vi "TL behavior obstacle avoidance.vi"(1 "Activate?":bool=TRUE, 2 "Sensor":cluster{"Name":string, "f":dbl}[](array[cluster])=[{"Name"="bow", "f"=20.0}, {"Name"="pbow", "f"=60.0}, {"Name"="port", "f"=0.0}, {"Name"="sbow", "f"=60.0}, {"Name"="starboard", "f"=0.0}]) -> (0 "Obs Avoid Array":dbl[](array[numeric]))   [LabVIEW 2013]
doc: "This vi uses the values from the Bow, PBow and SBow IR sensors to create an Obstacle Avoidance Array. The value range between 1 and -1."
panel:
  out "Waveform Graph":cluster{dbl, dbl, dbl[]}(graph)
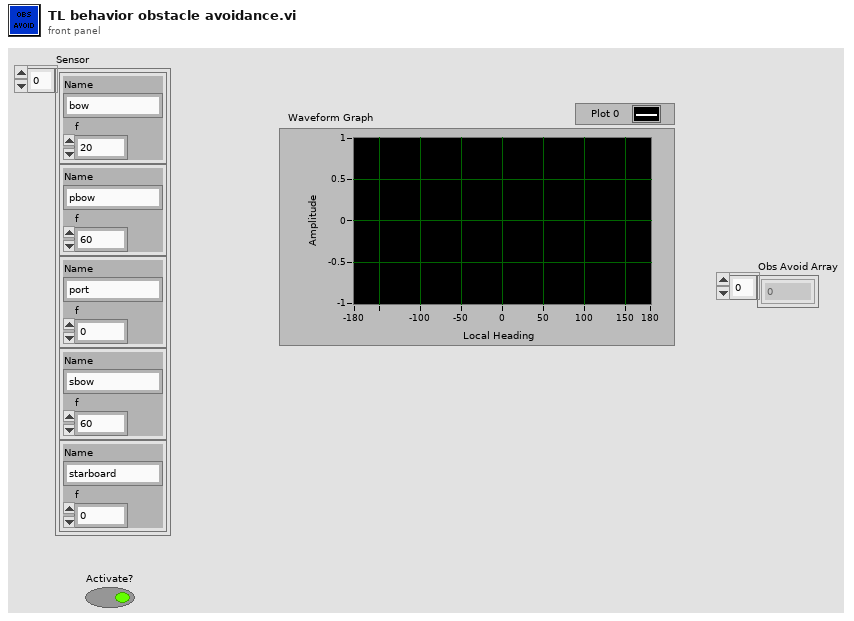
[diagram p1: front panel]
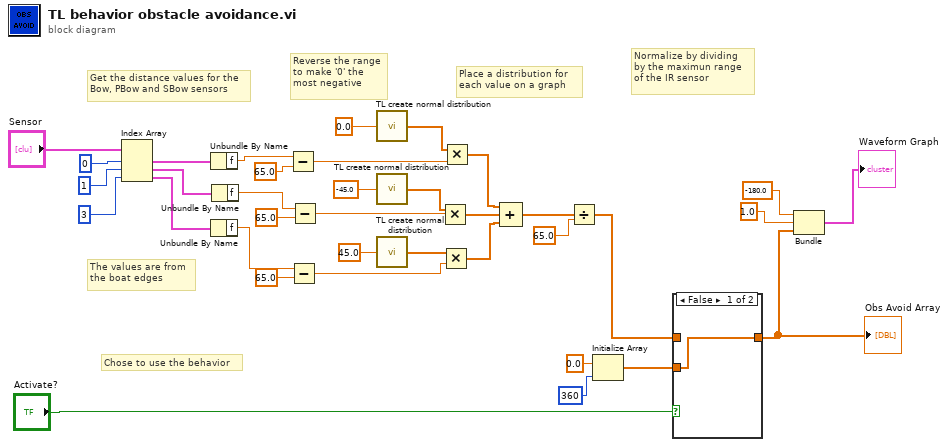
[diagram p0: block diagram]
diagram:
  # "Chose to use the behavior"
  # "Reverse the range\nto make '0' the\nmost negative"
  # "Normalize by dividing\nby the maximun range\nof the IR sensor"
  # "The values are from\nthe boat edges"
  # "Place a distribution for \neach value on a graph"
  # "Get the distance values for the\nBow, PBow and SBow sensors"
  n1 = Index Array(array="Sensor", index #1=0 ("index"), index #2=1 ("index"), index #3=3 ("index")) -> (element #1=w32:cluster{"Name":string, "f":dbl}, element #2=w31:cluster{"Name":string, "f":dbl}, element #3=w30:cluster{"Name":string, "f":dbl})
  n2 = Unbundle By Name(w32) -> ("f"=w15:dbl)
  n3 = Unbundle By Name(w30) -> ("f"=w12:dbl)
  n4 = Unbundle By Name(w31) -> ("f"=w10:dbl)
  n5 = Subtract(x=w15, y=65.0) -> (x-y=w9:dbl)
  n6 = Subtract(x=w12, y=65.0) -> (x-y=w7:dbl)
  n7 = Subtract(x=w10, y=65.0) -> (x-y=w8:dbl)
  n8 = call "TL create normal distribution.vi"("mean"=0.0) -> ("ACT array"=w23:dbl[])
  n9 = call "TL create normal distribution.vi"("mean"=-45.0) -> ("ACT array"=w22:dbl[])
  n10 = call "TL create normal distribution.vi"("mean"=45.0) -> ("ACT array"=w21:dbl[])
  n11 = Multiply(x=w22, y=w8) -> (x*y=w20:dbl[])
  n12 = Multiply(x=w21, y=w7) -> (x*y=w18:dbl[])
  n13 = Multiply(x=w23, y=w9) -> (x*y=w19:dbl[])
  n14 = Compound Arithmetic op=ADD(w19, w20, w18) -> (w17:dbl[])
  n15 = Divide(x=w17, y=65.0) -> (x/y=w2:dbl[])
  n16 = Initialize Array(0.0 ("element"), 360 ("dimension size")) -> (w3:dbl[])
  n17 = case shown="False" "Activate?" {
    tunnel: w2 -> [_ w38]
    tunnel: w3 -> [w37 _]
    tunnel: [w37 w38] -> w1
    frame False {
    }
    frame True {
    }
  }
  "Obs Avoid Array" <- w1
  n18 = Bundle(-180.0, 1.0, w1) -> (→"Waveform Graph":cluster{dbl, dbl, dbl[]})  [unwired: 1 in]
